vi "PDP Heater= Message.vi"(0 "Setrate":bool) -> ()   [LabVIEW 2009]
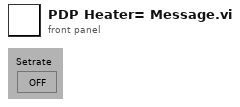
[diagram p1: front panel]
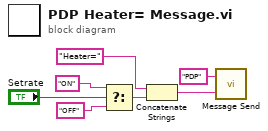
[diagram p0: block diagram]
diagram:
  n1 = Select(t="ON", s="Setrate", f="OFF") -> (s? t:f=w6:string)
  n2 = Concatenate Strings("Heater=" ("Substring"), w6) -> (w2:string)
  n3 = call "Message Send.vi"("Message"=w2, "Destination"="PDP") -> ()
